vi "TDMSAdv defragment .vi"(8 "error in (no error)":errorcluster, 10 "filePath":path, 11 "TDMSAdv in":refnum<class "TDMSAdv.lvclass">) -> (0 "error out":errorcluster, 3 "TDMSAdv out":refnum<class "TDMSAdv.lvclass">)   [LabVIEW 2018, in "TDMSAdv.lvclass"]
uses:
  TDMSAdv.lvclass
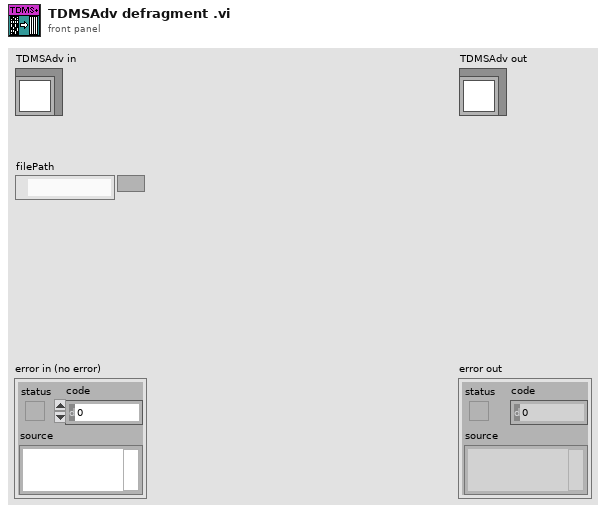
[diagram p1: front panel]
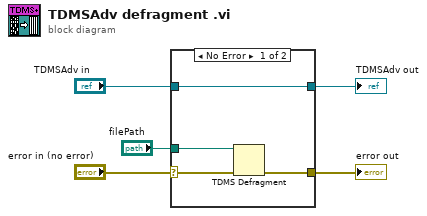
[diagram p0: block diagram]
diagram:
  n1 = case shown="No Error" "error in (no error)" {
    selector: "error in (no error)" -> [w6 w11]
    tunnel: [w7 w11] -> w4
    tunnel: [w8 w10] -> w2
    tunnel: "TDMSAdv in" -> [w8 w10]
    tunnel: "filePath" -> [w9 _]
    frame No Error {
      n2 = TDMS Defragment(4:w6, 7:w9) -> (0:w7:errorcluster)
    }
    frame Error {
    }
  }
  "error out" <- w4
  "TDMSAdv out" <- w2
